vi "Fill Stitch Lists.vi"(4 "error IN":errorcluster) -> (0 "error OUT":errorcluster)   [LabVIEW 2015]
uses:
  BIMS_Collector Globals.vi
panel:
  out "Query":string
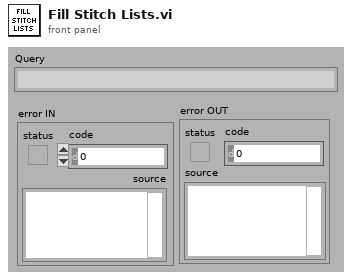
[diagram p1: front panel]
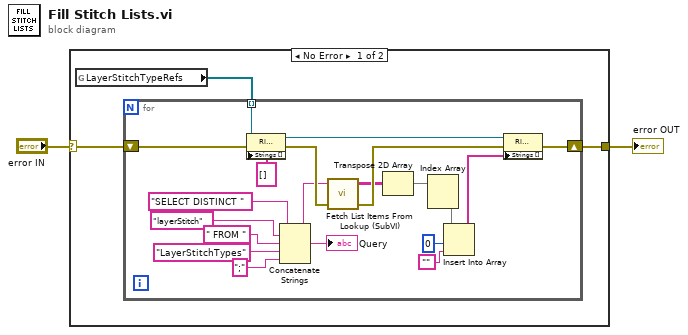
[diagram p0: block diagram]
diagram:
  n1 = case shown="No Error" "error IN" {
    selector: "error IN" -> [w4 w25]
    tunnel: [w5 w25] -> w1
    frame No Error {
      n2 = global read "BIMS_Collector Globals.vi" "LayerStitchTypeRefs"() -> (w3:refnum<vi>[])
      n3 = for {
        tunnel: w3 -> [w15] mode=indexing
        shift-right: [w23] -> w5
        shift-left: w4 -> [w12]
        n4 = property class="Ring (strict)"(reference=w15, error in=w12, "Strings []"=string[] []) -> (reference out=w14:refnum<vi>, error out=w13:errorcluster)
        n5 = Concatenate Strings("SELECT DISTINCT " ("string"), "layerStitch" ("Table"), " FROM " ("string"), "LayerStitchTypes" ("Table"), ";" ("string")) -> (w8:string)
        "Query" <- w8
        n6 = call "Fetch List Items From Lookup (SubVI).vi"("error IN"=w13, "Query"=w8) -> ("error OUT"=w24:errorcluster, "recordset data"=w18:string[][])  [unwired: 2 out]
        n7 = Transpose 2D Array(2D array=w18) -> (transposed array=w19:string[][])
        n8 = Index Array(array=w19) -> (element=w22:string[])  [unwired: 2 in]
        n9 = Insert Into Array "Insert Into Array"(array=w22, index=0, new element="" ("new element/subarray")) -> (w17:string[])
        n10 = property class="Ring (strict)"(reference=w14, error in=w24, "Strings []"=w17) -> (error out=w23:errorcluster)  [unwired: 1 out]
      }
    }
    frame Error {
    }
  }
  "error OUT" <- w1
